vi "AIT 1553 - Remove Bus.vi"(8 "error in (no error)":errorcluster, 10 "Bus":u16, 11 "Node Ptr":u64 format="%.0x") -> (0 "error out":errorcluster)   [LabVIEW 2013]
uses:
  Controls and Global/Global.vi
  <vilib>/NI Veristand/Custom Device API/Get Item Property (U16).vi
  AIT 664 Custom Device.lvlib
  <vilib>/NI Veristand/Custom Device Tools/Custom Device Utility Library/Custom Device Utility Library.lvlib
  <vilib>/NI Veristand/Custom Device API/Custom Device API.lvlib
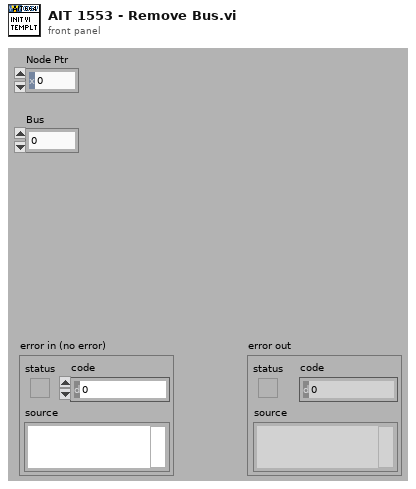
[diagram p1: front panel]
types:
  T1 = typedef "Custom Device API.lvlib/Custom Device Item Ref.ctl" = u64
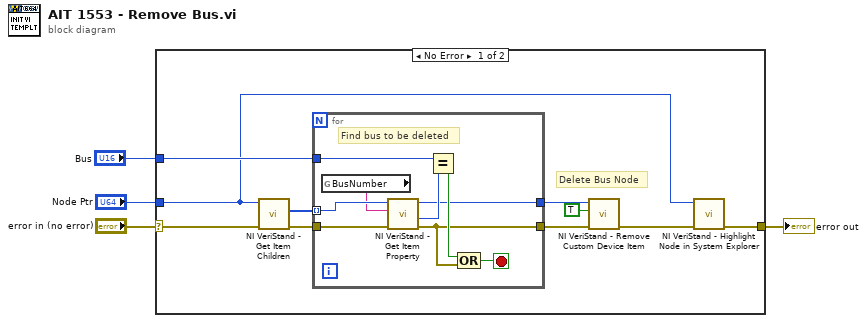
[diagram p0: block diagram]
diagram:
  n1 = case shown="No Error" "error in (no error)" {
    selector: "error in (no error)" -> [w14 w24]
    tunnel: "Node Ptr" -> [w6 _]
    tunnel: [w13 w24] -> w2
    tunnel: "Bus" -> [w10 _]
    frame No Error {
      # "Delete Bus Node"
      n2 = call <vilib>:"NI VeriStand - Get Item Children.vi"("error in (no error)"=w14, "Item Ref in"=w6) -> ("error out"=w11:errorcluster, "Child Refs"=w12:T1[])  [unwired: 6 in, 2 out]
      n3 = for {
        tunnel: w12 -> [w22] mode=indexing
        tunnel: w11 -> [w23]
        tunnel: w10 -> [w19]
        tunnel: [w16] -> w9
        tunnel: [w15] -> w8
        stop <- w17 stop-if-true
        # "Find bus to be deleted"
        n4 = global read "Global.vi" "BusNumber"() -> (w21:string)
        n5 = call-poly <vilib>:"NI VeriStand - Get Item Property.vi"("error in (no error)"=w23, "Property Name"=w21, "Item Ref in"=w22) -> ("error out"=w16:errorcluster, "Value"=w20:u16, "Item Ref out"=w15:T1)  [unwired: 5 in, 1 out]
        n6 = Equal?(x=w19, y=w20) -> (x = y?=w18:bool)
        n7 = Compound Arithmetic op=OR(w18, w16) -> (w17:bool)
      }
      n8 = call <vilib>:"NI VeriStand - Remove Custom Device Item.vi"("error in (no error)"=w9, "Force Delete (F)"=TRUE, "Item Ref in"=w8) -> ("error out"=w7:errorcluster)  [unwired: 7 in, 1 out]
      n9 = call <vilib>:"NI VeriStand - Highlight Node in System Explorer.vi"("error in (no error)"=w7, "Item Ref in"=w6) -> ("error out"=w13:errorcluster)  [unwired: 8 in, 1 out]
    }
    frame Error {
    }
  }
  "error out" <- w2
